vi "lab1MM.vi"() -> ()   [LabVIEW 2019]
panel:
  out "triangle":dbl(graph)
  out "square":dbl(graph)
  in  "stop":bool
  out "sine":dbl(graph)
  in  "offset":dbl
  in  "A":dbl
  in  "f":dbl
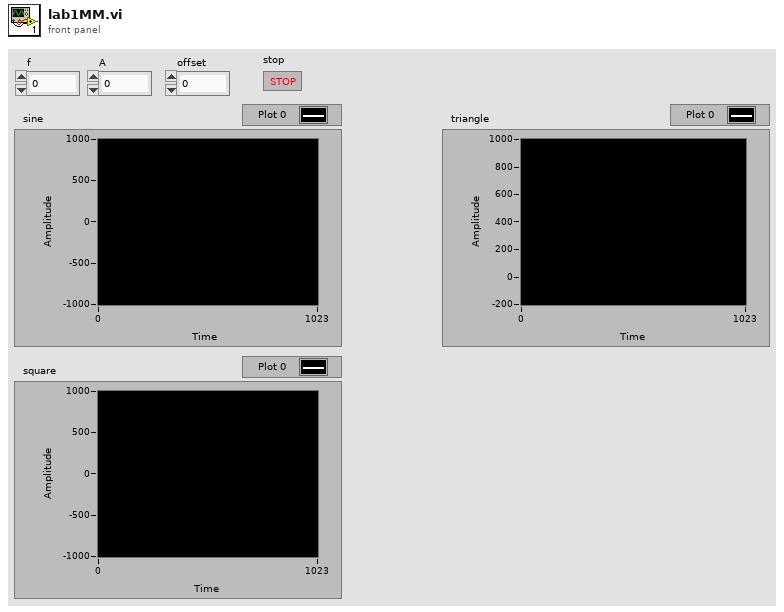
[diagram p1: front panel]
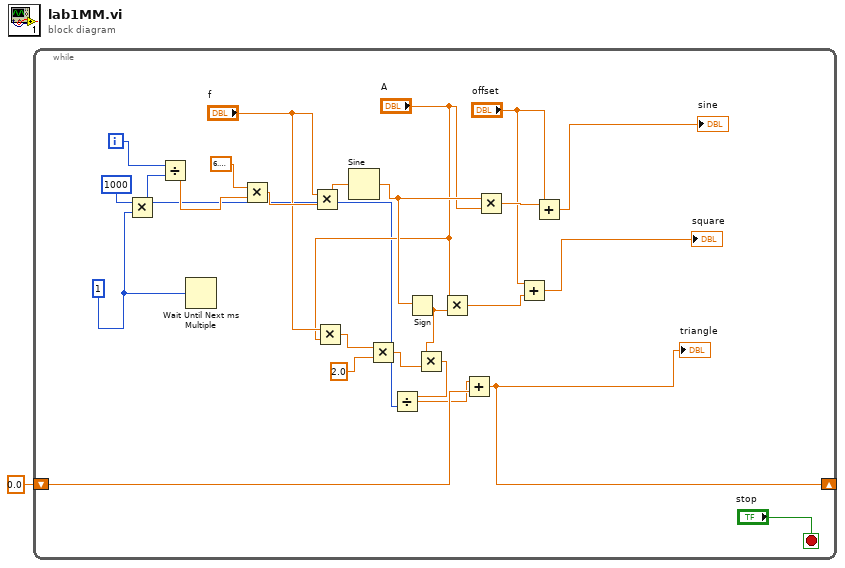
[diagram p0: block diagram]
diagram:
  n1 = while {
    shift-right: [w13] -> _
    shift-left: 0.0 -> [w12]
    i -> [w25]
    stop <- "stop" stop-if-true
    w20 = 1
    w4 = 1000
    n2 = Multiply(x=w4, y=w20) -> (x*y=w24:i32)
    n3 = Divide(x=w25, y=w24) -> (x/y=w11:dbl)
    n4 = Wait Until Next ms Multiple(millisecond multiple=w20) -> ()  [unwired: 1 out]
    n5 = Multiply(x=6.283185307179586, y=w11) -> (x*y=w22:dbl)
    n6 = Multiply(x="f", y=w22) -> (x*y=w23:dbl)
    n7 = Multiply(x="f", y="A") -> (x*y=w7:dbl)
    n8 = Sine(x=w23) -> (sin(x)=w17:dbl)
    n9 = Multiply(x=w7, y=2.0) -> (x*y=w5:dbl)
    n10 = Sign(1:w17) -> (0:w8:dbl)
    n11 = Multiply(x=w8, y=w5) -> (x*y=w3:dbl)
    n12 = Divide(x=w3, y=w4) -> (x/y=w2:dbl)
    n13 = Multiply(x="A", y=w8) -> (x*y=w15:dbl)
    n14 = Add(x=w2, y=w12) -> (x+y=w13:dbl)
    "triangle" <- w13
    n15 = Multiply(x=w17, y="A") -> (x*y=w19:dbl)
    n16 = Add(x="offset", y=w15) -> (x+y=→"square":dbl)
    n17 = Add(x=w19, y="offset") -> (x+y=→"sine":dbl)
  }
